vi "Delete.vi"(8 "Error In":errorcluster, 11 "LQCoreEngine in":refnum<class "LQCoreEngine.lvclass">) -> (0 "Error Out":errorcluster)   [LabVIEW 2014, in "LQ Core.lvlib" / "LQCoreEngine.lvclass"]
doc: "You cannot delete an LQ Engine! Call \"Stop Engine.vi\" instead."
uses:
  LQCoreEngine.lvclass
  <vilib>/Utility/error.llb/Error Cluster From Error Code.vi
  <vilib>/ErrorRing/Error Ring.xnode
panel:
  # "Copyright (c) 2021 Sze Howe Koh\n\nThis Source Code Form is subject to the terms of the Mozilla Public\nLicense, v. 2.0. If a copy of the MPL was not distributed with this\nfile, You can obtain one at http://mozilla.org/MPL/2.0/."
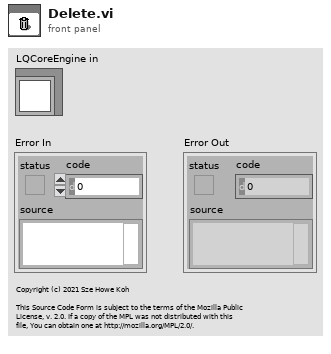
[diagram p1: front panel]
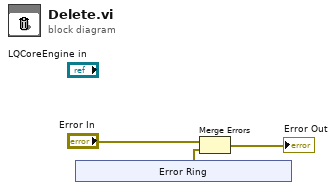
[diagram p0: block diagram]
diagram:
  n1 = xnode "Error Ring"() -> ("error out"=w3:errorcluster)
  n2 = Merge Errors("Error In", w3) -> (→"Error Out":errorcluster)
